vi "TankDrive.vi"(4 "AccelRate":dbl, 5 "Cutoff":dbl=0.15 format="%#_13g", 6 "LoopTime":dbl, 7 "DriveAction":T9, 8 "error in (no error)":errorcluster, 9 "RightDesired":dbl, 10 "LeftDesired":dbl, 11 "RobotDriveDevRef":T1={"DevStatus"={"status"=FALSE, "code"=0, "source"=""}, "Motors[]"=[], "Square Inputs"=FALSE, "Max Output"=1.0, "Isochronous"=FALSE}) -> (0 "error out":errorcluster)   [LabVIEW 2013]
doc: "TankDrive has the following actions:\n-Init: takes a motor reference and stores it in a shift register, so you only need to pass the rerference once.\n-SetValue: sets the motor values directly, no processing involved.\n-LinearDrive: uses the loop time, acceleration rate, and cutoff to avoid reaching the desired input. The loop time and acceleration rate determine the max change in motor input that is allowed. The cutoff is the minimum motor input; if the desired value is greater than the cutoff, then the current motor input will at least be bumped up to the cutoff.\n-Disabled: turns the motors off."
uses:
  TankDriveAction.ctl
  <vilib>/Rock Robotics/WPI/RobotDrive/WPI_RobotDriveDevRef.ctl
  <vilib>/Rock Robotics/WPI/MotorControl/WPI_MotorControlDeviceRef.ctl
  <vilib>/Rock Robotics/SystemInterfaces/Typedef/FPGA_TypedefDigitalModule.ctl
  <vilib>/Rock Robotics/SystemInterfaces/DIO/FPGA_DIOPWMChannel.ctl
  <vilib>/Rock Robotics/WPI/PWM/WPI_PWMDeadband.ctl
  <vilib>/Rock Robotics/WPI/CAN/Jaguar/SubVIs/WPI_CANJaguar_ControlMode.ctl
  <vilib>/Rock Robotics/WPI/PWM/WPI_PWMTransform_ConPane.ctl
panel:
  in  "Skip":dbl=1.5
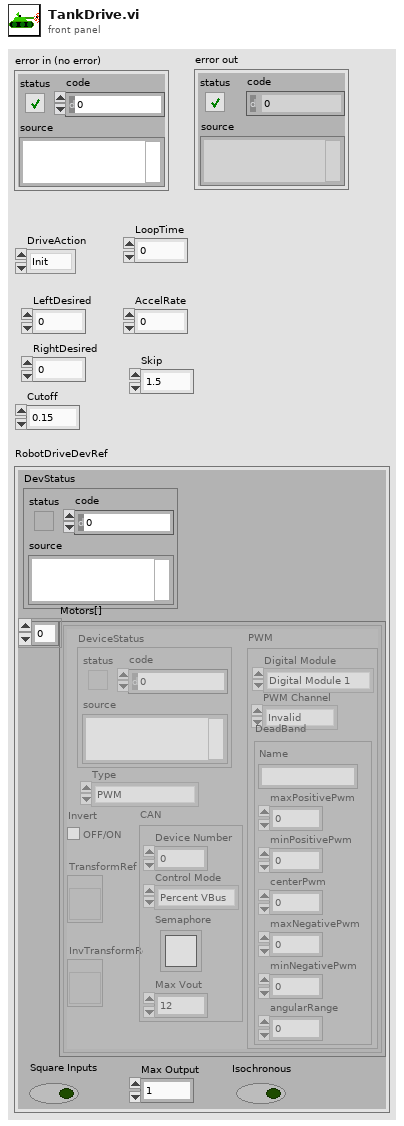
[diagram p1: front panel]
types:
  T1 = typedef "WPI_RobotDriveDevRef.ctl" = cluster{"DevStatus":errorcluster, "Motors[]":T2[], "Square Inputs":bool, "Max Output":dbl, "Isochronous":bool}
  T2 = typedef "WPI_MotorControlDeviceRef.ctl" = cluster{"DeviceStatus":errorcluster, "Type":enum16{"PWM", "CAN"}, "PWM":cluster{"Digital Module":T3, "PWM Channel":T4, "DeadBand":T5}, "CAN":cluster{"Device Number":u8, "Control Mode":T6, "Semaphore":T7, "Max Vout":dbl}, "Invert":bool, "TransformRef":T8, "InvTransformRef":T8}
  T3 = typedef "FPGA_TypedefDigitalModule.ctl" = enum16{"Digital Module 1", "Digital Module 2"}
  T4 = typedef "FPGA_DIOPWMChannel.ctl" = enum8{"PWM 1", "PWM 2", "PWM 3", "PWM 4", "PWM 5", "PWM 6", "PWM 7", "PWM 8", "PWM 9", "PWM 10", "Invalid"}
  T5 = typedef "WPI_PWMDeadband.ctl" = cluster{"Name":string, "maxPositivePwm":i32, "minPositivePwm":i32, "centerPwm":i32, "maxNegativePwm":i32, "minNegativePwm":i32, "angularRange":u16}
  T6 = typedef "WPI_CANJaguar_ControlMode.ctl" = enum8{"Percent VBus", "Current", "Speed", "Position", "Voltage"}
  T7 = typedef "Semaphore RefNum" = refnum<k1>
  T8 = typedef "WPI_PWMTransform_ConPane.ctl" = refnum<vi>
  T9 = typedef "TankDriveAction.ctl" = enum16{"Init", "LinearDrive", "SetValue", "Disable"}
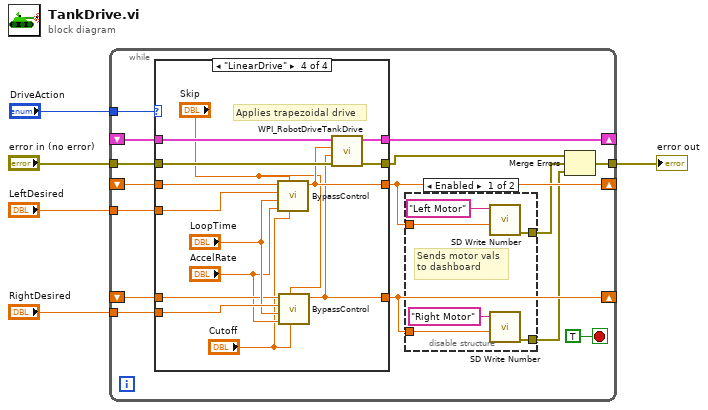
[diagram p0: block diagram]
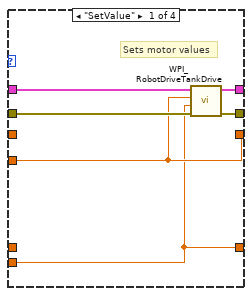
[diagram p3: hidden frame]
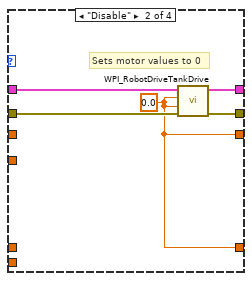
[diagram p4: hidden frame]
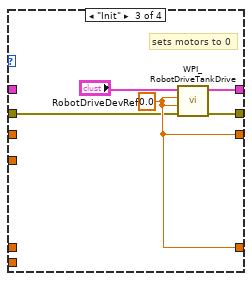
[diagram p5: hidden frame]
diagram:
  n1 = while {
    shift-right: [w20] -> _
    shift-left: _ -> [w18]
    tunnel: "error in (no error)" -> [w17]
    tunnel: "DriveAction" -> [w16]
    tunnel: "LeftDesired" -> [w15]
    tunnel: "RightDesired" -> [w14]
    shift-right: [w12] -> _
    shift-left: _ -> [w13]
    shift-right: [w11] -> _
    shift-left: _ -> [w10]
    tunnel: [w9] -> w1
    stop <- TRUE stop-if-true
    n2 = case shown="\"LinearDrive\"" w16 {
      tunnel: [w27 w36 w40 w49] -> w20
      tunnel: w18 -> [w28 w37 _ w48]
      tunnel: w17 -> [w32 w35 w38 w55]
      tunnel: [w31 w34 w42 w56] -> w8
      tunnel: [w30 w33 w41 w52] -> w12
      tunnel: [w29 w33 w41 w51] -> w11
      tunnel: w15 -> [w30 _ _ w54]
      tunnel: w14 -> [w29 _ _ w53]
      tunnel: w13 -> [_ _ _ w47]
      tunnel: w10 -> [_ _ _ w46]
      frame "SetValue" {
        # "Sets motor values"
        n3 = call <vilib>:"WPI_RobotDriveTankDrive.vi"("error in (no error)"=w32, "Right axis value"=w29, "Left axis value"=w30, "RobotDriveDevRef"=w28) -> ("error out"=w31:errorcluster, "RobotDriveDevRef"=w27:T1)  [unwired: 5 in, 1 out]
      }
      frame "Disable" {
        w33 = 0.0
        # "Sets motor values to 0"
        n4 = call <vilib>:"WPI_RobotDriveTankDrive.vi"("error in (no error)"=w35, "Right axis value"=w33, "Left axis value"=w33, "RobotDriveDevRef"=w37) -> ("error out"=w34:errorcluster, "RobotDriveDevRef"=w36:T1)  [unwired: 5 in, 1 out]
      }
      frame "Init" {
        w41 = 0.0
        # "sets motors to 0"
        n5 = call <vilib>:"WPI_RobotDriveTankDrive.vi"("error in (no error)"=w38, "Right axis value"=w41, "Left axis value"=w41, "RobotDriveDevRef"="RobotDriveDevRef") -> ("error out"=w42:errorcluster, "RobotDriveDevRef"=w40:T1)  [unwired: 5 in, 1 out]
      }
      frame "LinearDrive" {
        # "Applies trapezoidal drive"
        n6 = call "BypassControl.vi"("Cutoff"="Cutoff", "Skip"="Skip", "AccelRate"="AccelRate", "LoopTime"="LoopTime", "DesiredInput"=w54, "CurrentInput"=w47) -> ("SetMotor"=w52:dbl)  [unwired: 5 in]
        n7 = call "BypassControl.vi"("Cutoff"="Cutoff", "Skip"="Skip", "AccelRate"="AccelRate", "LoopTime"="LoopTime", "DesiredInput"=w53, "CurrentInput"=w46) -> ("SetMotor"=w51:dbl)  [unwired: 5 in]
        n8 = call <vilib>:"WPI_RobotDriveTankDrive.vi"("error in (no error)"=w55, "Right axis value"=w51, "Left axis value"=w52, "RobotDriveDevRef"=w48) -> ("error out"=w56:errorcluster, "RobotDriveDevRef"=w49:T1)  [unwired: 5 in, 1 out]
      }
    }
    n9 = disable-structure shown="Enabled" {
      disable-tunnel: w12 -> [w24 _]
      disable-tunnel: w11 -> [w23 _]
      disable-tunnel: [w22 _] -> w7
      disable-tunnel: [w21 _] -> w6
      frame Enabled {
        # "Sends motor vals\nto dashboard"
        n10 = call <vilib>:"SD Write Number.vi"("Numeric"=w24, "Name"="Left Motor") -> ("error out"=w22:errorcluster)  [unwired: 8 in, 1 out]
        n11 = call <vilib>:"SD Write Number.vi"("Numeric"=w23, "Name"="Right Motor") -> ("error out"=w21:errorcluster)  [unwired: 8 in, 1 out]
      }
      frame Disabled {
      }
    }
    n12 = Merge Errors(w8, w7, w6) -> (w9:errorcluster)
  }
  "error out" <- w1
